vi "HEWH Check for Uninitialized Dates.vi"(10 "date string":string, 11 "Elapsed days in":i32) -> (3 "Elapsed days out":i32)   [LabVIEW 2014]
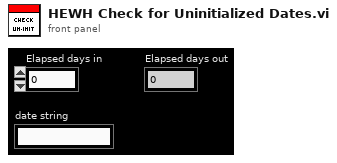
[diagram p1: front panel]
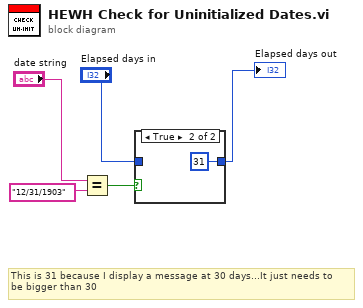
[diagram p0: block diagram]
diagram:
  # "This is 31 because I display a message at 30 days...It just needs to \nbe bigger than 30"
  n1 = Equal?(x="date string", y="12/31/1903" ("date string 2")) -> (x = y?=w3:bool)
  n2 = case shown="True" w3 {
    tunnel: "Elapsed days in" -> [w6 _]
    tunnel: [w6 31 ("Elapsed days")] -> w5
    frame False {
    }
    frame True {
    }
  }
  "Elapsed days out" <- w5
